vi "TEST Report Class.vi"() -> ()   [LabVIEW 2011]
doc: "This is a very simple VI to test the functionality of any child to the Report class. Specifically it is used to test the LVOOP exercise.\n\nAAL 9/09"
uses:
  Plug Ins/TXT Report Class/TXT Report.lvclass
panel:
  in  "Header":string="Rocky Mountain High...   Colorado..."
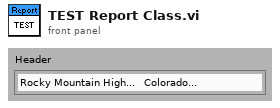
[diagram p1: front panel]
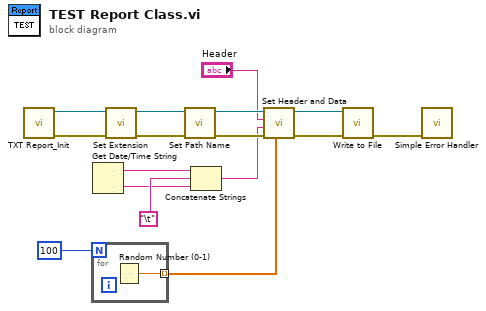
[diagram p0: block diagram]
diagram:
  n1 = call "TXT Report_Init.vi"() -> ("error out"=w1:errorcluster, "TXT_Report out"=w2:refnum<class "TXT Report.lvclass">)  [unwired: 10 in]
  n2 = for {
    N: 100 -> [_]
    tunnel: [w17] -> w6 mode=indexing
    n3 = Random Number (0-1)() -> (number: 0 to 1=w17:dbl)
  }
  n4 = Get Date/Time String() -> (date string=w16:string, time string=w14:string)  [unwired: 3 out]
  n5 = call-dynamic "Set Extension.vi"("error in (no error)"=w1, "TXT_Report"=w2) -> ("error out"=w11:errorcluster, "TXT_Report out"=w12:refnum<class "TXT Report.lvclass">)  [unwired: 8 in]
  n6 = call-dynamic "Set Path Name.vi"("error in (no error)"=w11, "Report"=w12) -> ("error out"=w9:errorcluster, "Report out"=w10:refnum<class "TXT Report.lvclass">)  [unwired: 8 in]
  n7 = Concatenate Strings(w16, "\t", w14) -> (w7:string)
  n8 = call-dynamic "Set Header and Data.vi"("Data Array"=w6, "error in (no error)"=w9, "Data & Time String"=w7, "Header"="Header", "Report"=w10) -> ("error out"=w4:errorcluster, "Report out"=w5:refnum<class "TXT Report.lvclass">)  [unwired: 5 in]
  n9 = call-dynamic "Write to File.vi"("error in (no error)"=w4, "TXT Report"=w5) -> ("error out"=w3:errorcluster)  [unwired: 8 in, 1 out]
  n10 = call <vilib>:"Simple Error Handler.vi"("error in (no error)"=w3) -> ()  [unwired: 1 in, 8 out]
